vi "OLD Chroma 1905x Series System Error.vi"(8 "error in (no error)":errorcluster, 11 "VISA resource name":refnum<visa-resource-name>) -> (0 "error out":errorcluster, 2 "System Error":string, 3 "VISA resource name out":refnum<visa-resource-name>)   [LabVIEW 2025]
doc: "Chroma\n5 Clock Tower Place Suite 210\nMaynard, MA 01754\nTel: 1 800 253-1230\nTel: 1 877 4 A HIPOT\nFax: 1 978-461-4295\nWebsite: www.chroma.com"
uses:
  <instrlib>/Chroma 19052/Chroma 19052.lvlib
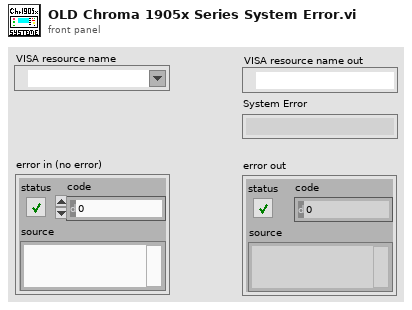
[diagram p1: front panel]
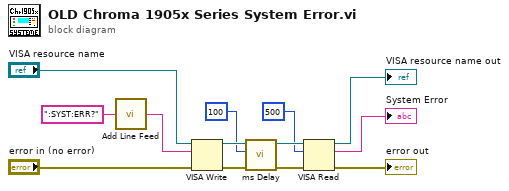
[diagram p0: block diagram]
diagram:
  n1 = call <instrlib>:"Add Line Feed.vi"("Command string"=":SYST:ERR?") -> ("Concatenated string"=w8:string)  [unwired: 4 in]
  n2 = VISA Write(VISA resource name="VISA resource name", write buffer=w8, error in (no error)="error in (no error)") -> (VISA resource name out=w12:refnum<visa-resource-name>, error out=w5:errorcluster)  [unwired: 1 out]
  n3 = call <instrlib>:"ms Delay.vi"("error in (no error)"=w5, "Time Delay [ms]"=u32 100 ("Time Delay S"), "VISA resource name"=w12) -> ("error out"=w7:errorcluster, "VISA resource name 2"=w13:refnum<visa-resource-name>)  [unwired: 7 in]
  n4 = VISA Read(VISA resource name=w13, byte count=u32 500 ("byte count (0)"), error in (no error)=w7) -> (VISA resource name out=→"VISA resource name out":refnum<visa-resource-name>, read buffer=→"System Error":string, error out=→"error out":errorcluster)  [unwired: 1 out]
